vi "Configure Digital Voltmeter.vi"(6 "DVM Type (0: Root-mean-square, without DC)":i32(ring) items=["Root-mean-square, without DC", "DC Value", "Root-mean-square", "Frequency Counter"], 7 "Enable DVM Analysis (F: Disable)":bool, 8 "error in (no error)":errorcluster, 9 "Auto Range (F: Disable)":bool, 10 "DVM Channel (1: Channel 1)":i32(ring)=1 items=["Channel 1"=1, "Channel 2"=2, "Channel 3"=3, "Channel 4"=4], 11 "VISA resource name":refnum<visa-resource-name>) -> (0 "error out":errorcluster, 3 "VISA resource name out":refnum<visa-resource-name>)   [LabVIEW 2017, in "Agilent 2000 3000 X-Series.lvlib"]
doc: "Controls the digital voltmeter (DVM) feature.\n\n<B>Note(s):</B>\nTo use this VI, the optional DSOXDVM digital voltmeter analysis feature must be licensed."
uses:
  Agilent 2000 3000 X-Series.lvlib
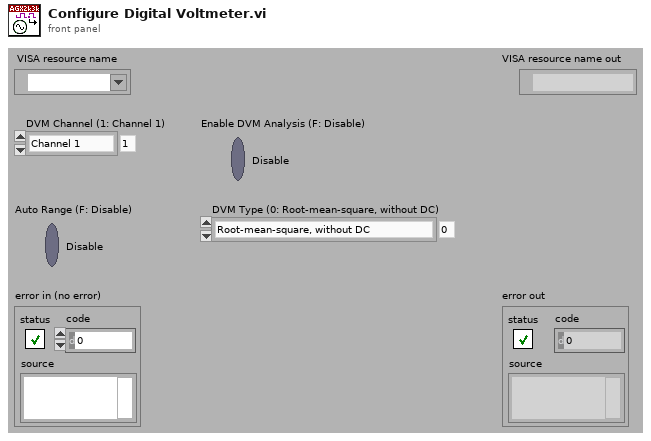
[diagram p1: front panel]
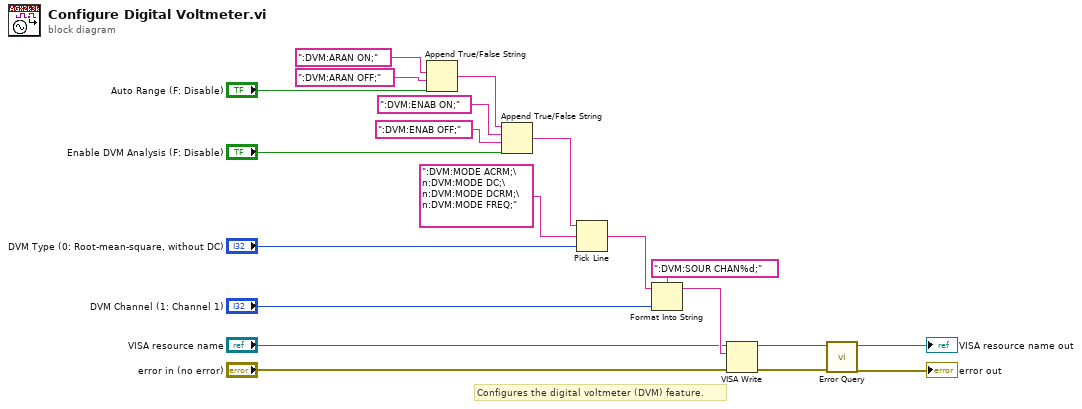
[diagram p0: block diagram]
diagram:
  # "Configures the digital voltmeter (DVM) feature."
  n1 = Append True/False String(1:"Auto Range (F: Disable)", 2:":DVM:ARAN OFF;", 3:":DVM:ARAN ON;") -> (0:w17:string)  [unwired: 1 out]
  n2 = Append True/False String(1:"Enable DVM Analysis (F: Disable)", 2:":DVM:ENAB OFF;", 3:":DVM:ENAB ON;", 4:w17) -> (0:w11:string)
  n3 = Pick Line(string ("")=w11, multi-line string=":DVM:MODE ACRM;\n:DVM:MODE DC;\n:DVM:MODE DCRM;\n:DVM:MODE FREQ;", line index="DVM Type (0: Root-mean-square, without DC)") -> (output string=w10:string)
  n4 = Format Into String(format string=":DVM:SOUR CHAN%d;", initial string=w10, "DVM Channel (1: Channel 1)") -> (resulting string=w7:string)  [unwired: 1 in, 1 out]
  n5 = VISA Write(VISA resource name="VISA resource name", write buffer=w7, error in (no error)="error in (no error)") -> (VISA resource name out=w4:refnum<visa-resource-name>, error out=w3:errorcluster)  [unwired: 1 out]
  n6 = call "Error Query.vi"("error in (no error)"=w3, "VISA resource name"=w4) -> ("error out"=→"error out":errorcluster, "VISA resource name out"=→"VISA resource name out":refnum<visa-resource-name>)  [unwired: 8 out]
